vi "PulseGenEPTx_5Inj_build.vi"(0 "PlsGenConfig":T2) -> (14 "OneShotArray":T1[](array[typedef]), 19 "Command Seq Output":T3)   [LabVIEW 2015, in "ECS-FPGA.lvlib"]
doc: "Builds ContinueSeq, CmdLevel, and Duration arrays for the command sequence block from the channel configuration control."
uses:
  <vilib>/Powertrain Controls/Device Drivers/Engine Position Tracking/EPTx/RevA/FPGA/Controls/EPTxAOSControl.ctl
  ECS-FPGA.lvlib
  <vilib>/Powertrain Controls/Device Drivers/Engine Position Tracking/EPTx/RevA/FPGA/EPTx - RevA - FPGA.lvlib
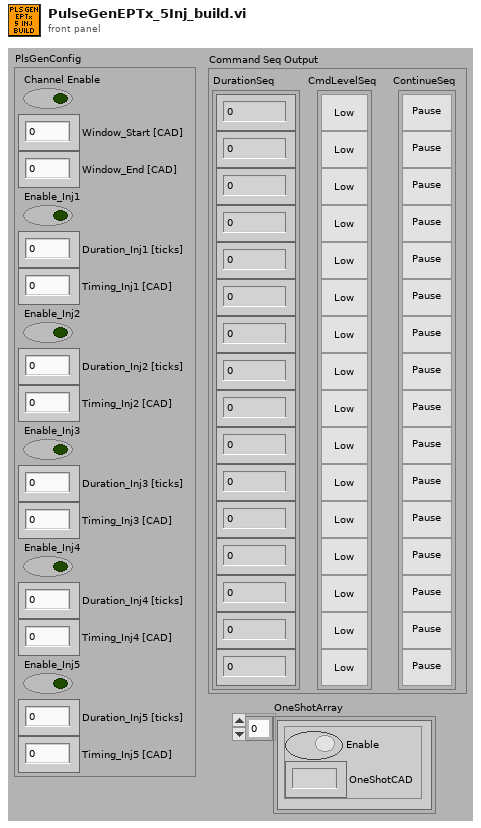
[diagram p1: front panel]
types:
  T1 = typedef "EPTx - RevA - FPGA.lvlib/EPTxAOSControl.ctl" = cluster{"Enable":bool, "OneShotCAD":fxp<+,18,11>}
  T2 = cluster{"Channel Enable":bool, "Window_Start [CAD]":fxp<+,18,11>, "Window_End [CAD]":fxp<+,18,11>, "Enable_Inj1":bool, "Duration_Inj1 [ticks]":u32, "Timing_Inj1 [CAD]":fxp<+,18,11>, "Enable_Inj2":bool, "Duration_Inj2 [ticks]":u32, "Timing_Inj2 [CAD]":fxp<+,18,11>, "Enable_Inj3":bool, "Duration_Inj3 [ticks]":u32, "Timing_Inj3 [CAD]":fxp<+,18,11>, "Enable_Inj4":bool, "Duration_Inj4 [ticks]":u32, "Timing_Inj4 [CAD]":fxp<+,18,11>, "Enable_Inj5":bool, "Duration_Inj5 [ticks]":u32, "Timing_Inj5 [CAD]":fxp<+,18,11>}
  T3 = cluster{"DurationSeq":u32[], "CmdLevelSeq":bool[], "ContinueSeq":bool[]}
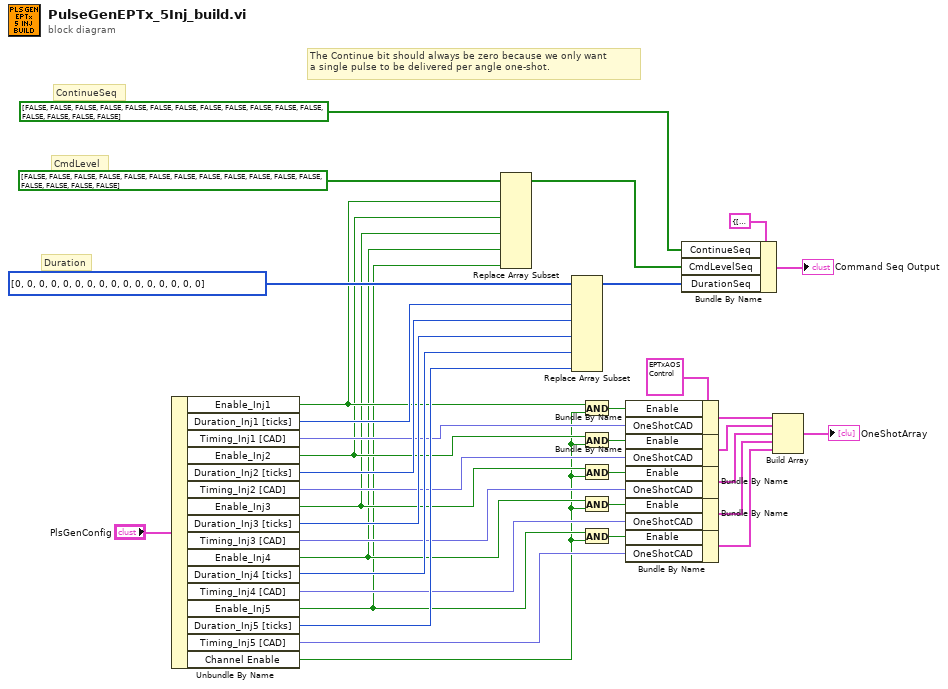
[diagram p0: block diagram]
diagram:
  w18 = T1 {"Enable"=FALSE, "OneShotCAD"=0.0} ("AOSControl")
  # "ContinueSeq"
  # "The Continue bit should always be zero because we only want \na single pulse to be delivered per angle one-shot."
  # "Duration"
  # "CmdLevel"
  n1 = Unbundle By Name("PlsGenConfig") -> ("Enable_Inj1"=w9:bool, "Duration_Inj1 [ticks]"=w36:u32, "Timing_Inj1 [CAD]"=w17:fxp<+,18,11>, "Enable_Inj2"=w8:bool, "Duration_Inj2 [ticks]"=w35:u32, "Timing_Inj2 [CAD]"=w16:fxp<+,18,11>, "Enable_Inj3"=w7:bool, "Duration_Inj3 [ticks]"=w34:u32, "Timing_Inj3 [CAD]"=w15:fxp<+,18,11>, "Enable_Inj4"=w4:bool, "Duration_Inj4 [ticks]"=w33:u32, "Timing_Inj4 [CAD]"=w14:fxp<+,18,11>, "Enable_Inj5"=w3:bool, "Duration_Inj5 [ticks]"=w32:u32, "Timing_Inj5 [CAD]"=w13:fxp<+,18,11>, "Channel Enable"=w2:bool)
  n2 = Replace Array Subset(array=bool[] [FALSE, FALSE, FALSE, FALSE, FALSE, FALSE, FALSE, FALSE, FALSE, FALSE, FALSE, FALSE, FALSE, FALSE, FALSE, FALSE] ("CmdLevelSeq"), new element #1=w9, new element #2=w8, new element #3=w7, new element #4=w4, new element #5=w3) -> (w27:bool[])  [unwired: 5 in]
  n3 = Replace Array Subset(array=u32[] [0, 0, 0, 0, 0, 0, 0, 0, 0, 0, 0, 0, 0, 0, 0, 0] ("DurationSeq"), new element #1=w36, new element #2=w35, new element #3=w34, new element #4=w33, new element #5=w32) -> (w28:u32[])  [unwired: 5 in]
  n4 = And(x=w9, y=w2) -> (x .and. y?=w12:bool)
  n5 = And(x=w8, y=w2) -> (x .and. y?=w11:bool)
  n6 = And(x=w7, y=w2) -> (x .and. y?=w10:bool)
  n7 = And(x=w4, y=w2) -> (x .and. y?=w6:bool)
  n8 = And(x=w3, y=w2) -> (x .and. y?=w5:bool)
  n9 = Bundle By Name(cluster=w18, "Enable"=w12, "OneShotCAD"=w17) -> (w19:T1)
  n10 = Bundle By Name(cluster=w18, "Enable"=w11, "OneShotCAD"=w16) -> (w20:T1)
  n11 = Bundle By Name(cluster=w18, "Enable"=w10, "OneShotCAD"=w15) -> (w21:T1)
  n12 = Bundle By Name(cluster=w18, "Enable"=w6, "OneShotCAD"=w14) -> (w22:T1)
  n13 = Bundle By Name(cluster=w18, "Enable"=w5, "OneShotCAD"=w13) -> (w23:T1)
  n14 = Bundle By Name(cluster=T3 {"DurationSeq"=[0, 0, 0, 0, 0, 0, 0, 0, 0, 0, 0, 0, 0, 0, 0, 0], "CmdLevelSeq"=[FALSE, FALSE, FALSE, FALSE, FALSE, FALSE, FALSE, FALSE, FALSE, FALSE, FALSE, FALSE, FALSE, FALSE, FALSE, FALSE], "ContinueSeq"=[FALSE, FALSE, FALSE, FALSE, FALSE, FALSE, FALSE, FALSE, FALSE, FALSE, FALSE, FALSE, FALSE, FALSE, FALSE, FALSE]} ("Command Seq Output"), "ContinueSeq"=bool[] [FALSE, FALSE, FALSE, FALSE, FALSE, FALSE, FALSE, FALSE, FALSE, FALSE, FALSE, FALSE, FALSE, FALSE, FALSE, FALSE], "CmdLevelSeq"=w27, "DurationSeq"=w28) -> (→"Command Seq Output":T3)
  n15 = Build Array(w19, w20, w21, w22, w23) -> (→"OneShotArray":T1[])
